vi "Handle Message.vi"(5 "Stack ID":u8, 7 "Function ID":u8, 8 "error in (no error)":errorcluster, 10 "Data":string, 11 "IO-4 Bricklet in":refnum<class "IO-4 Bricklet.lvclass">) -> (0 "error out":errorcluster, 1 "Send Answer":bool, 2 "Answer":variant, 3 "IO-4 Bricklet out":refnum<class "IO-4 Bricklet.lvclass">)   [LabVIEW 2011, in "Tinkerforge.lvlib" / "IO-4 Bricklet.lvclass"]
doc: "This VI is the child implementation of \"Handle Message.vi\" and processes all responses for this device type."
uses:
  IO-4 Bricklet.lvclass
  Type Definitions/Configuration.ctl
  Type Definitions/Interrupt.ctl
  IO-4 Bricklet.lvclass/IO-4 Bricklet.ctl
  Device/Device.lvclass
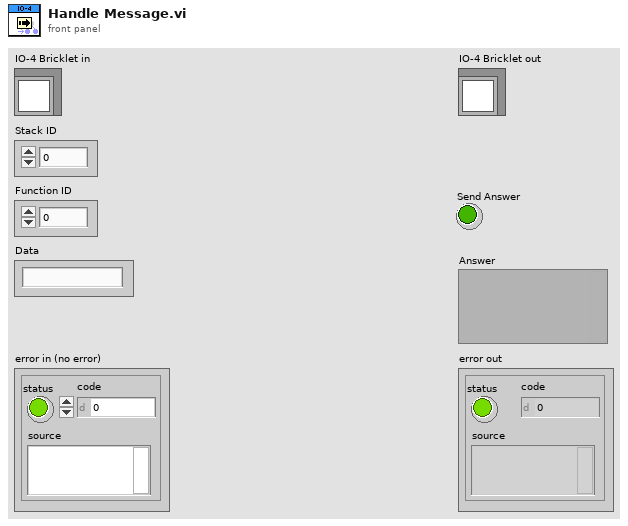
[diagram p1: front panel]
types:
  T1 = typedef "Tinkerforge.lvlib/IO-4 Bricklet.lvclass/Configuration.ctl" = cluster{"Direction Mask":u8, "Value Mask":u8}
  T2 = typedef "Tinkerforge.lvlib/IO-4 Bricklet.lvclass/Interrupt.ctl" = cluster{"Interrupt Mask":u8, "Value Mask":u8}
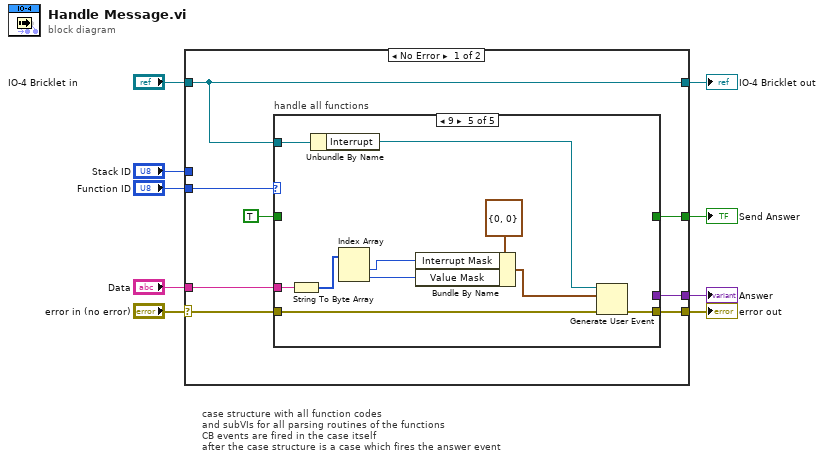
[diagram p0: block diagram]
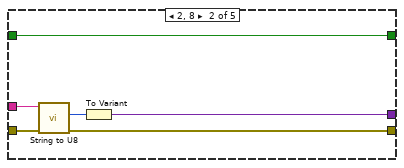
[diagram p3: hidden frame]
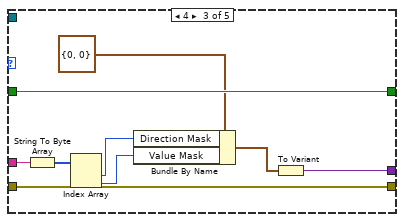
[diagram p4: hidden frame]
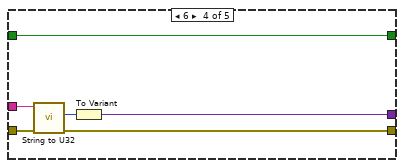
[diagram p5: hidden frame]
diagram:
  # "case structure with all function codes\nand subVIs for all parsing routines of the functions\nCB events are fired in the case itself\nafter the case structure is a case which fires the answer event"
  n1 = case shown="No Error" "error in (no error)" {
    selector: "error in (no error)" -> [w14 w49]
    tunnel: "IO-4 Bricklet in" -> [w17 w50]
    tunnel: "Stack ID" -> [_ _]
    tunnel: "Function ID" -> [w16 _]
    tunnel: "Data" -> [w13 _]
    tunnel: [w17 w50] -> w4
    tunnel: [w12 w49] -> w3
    tunnel: [w11 _] -> w2
    tunnel: [w10 _] -> w1
    frame No Error {
      n2 = case "handle all functions" shown="9" w16 {
        tunnel: w14 -> [_ w21 w28 w36 w40]
        tunnel: TRUE -> [_ w23 w32 w38 _]
        tunnel: [_ w23 w32 w38 _] -> w10
        tunnel: [_ w19 w28 w34 w46] -> w12
        tunnel: [_ w22 w31 w37 _] -> w11
        tunnel: w17 -> [_ _ _ _ w48]
        tunnel: w13 -> [_ w20 w30 w35 w45]
        frame Default {
          # "nothing to do"
        }
        frame 2, 8 {
          n3 = call "String to U8.vi"("Error In"=w21, "String"=w20) -> ("Error Out"=w19:errorcluster, "U8"=w18:u8)  [unwired: 7 in, 1 out]
          n4 = To Variant(anything=w18) -> (Variant=w22:variant)
        }
        frame 4 {
          n5 = String To Byte Array(string=w30) -> (unsigned byte array=w29:u8[])
          n6 = Index Array(array=w29) -> (element #1=w26:u8, element #2=w25:u8)  [unwired: 2 in]
          n7 = Bundle By Name(cluster=T1 {"Direction Mask"=0, "Value Mask"=0} ("Configuration"), "Direction Mask"=w26, "Value Mask"=w25) -> (w24:T1)
          n8 = To Variant(anything=w24) -> (Variant=w31:variant)
        }
        frame 6 {
          n9 = call "String to U32.vi"("Error In"=w36, "String"=w35) -> ("Error Out"=w34:errorcluster, "U32"=w33:u32)  [unwired: 7 in, 1 out]
          n10 = To Variant(anything=w33) -> (Variant=w37:variant)
        }
        frame 9 {
          n11 = String To Byte Array(string=w45) -> (unsigned byte array=w44:u8[])
          n12 = Unbundle By Name(w48) -> ("Interrupt"=w47:refnum<user-event>)
          n13 = Index Array(array=w44) -> (element #1=w41:u8, element #2=w42:u8)  [unwired: 2 in]
          n14 = Bundle By Name(cluster=T2 {"Interrupt Mask"=0, "Value Mask"=0} ("Interrupt"), "Interrupt Mask"=w41, "Value Mask"=w42) -> (w39:T2)
          n15 = Generate User Event(user event=w47, event data cluster=w39, error in=w40) -> (error out=w46:errorcluster)  [unwired: 1 out]
        }
      }
    }
    frame Error {
    }
  }
  "error out" <- w3
  "IO-4 Bricklet out" <- w4
  "Answer" <- w2
  "Send Answer" <- w1
